vi "CRYSet Graph Title.vi"(8 "Inserted Graph VIRef out":refnum<vi>, 9 "Frame VIRef":refnum<vi>, 10 "Title State":bool, 11 "Title Name in":string) -> (3 "Title Name out":string)   [LabVIEW 2013]
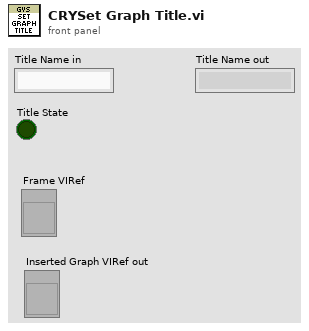
[diagram p1: front panel]
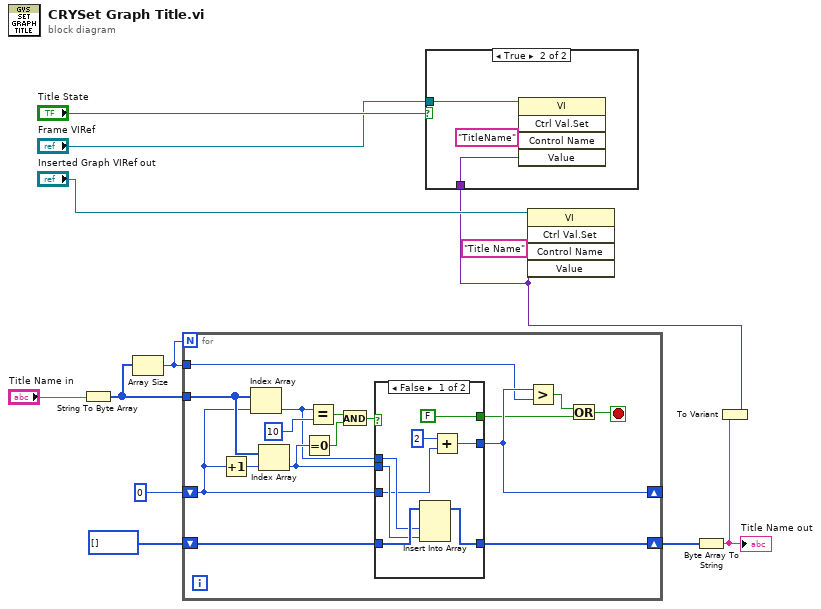
[diagram p0: block diagram]
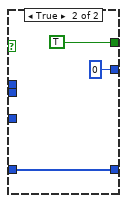
[diagram p3: hidden frame]
diagram:
  n1 = String To Byte Array(string="Title Name in") -> (unsigned byte array=w11:u8[])
  n2 = Array Size(array=w11) -> (size(s)=w9:i32)
  n3 = for {
    N: w9 -> [_]
    tunnel: w11 -> [w27]
    shift-right: [w19] -> w8
    shift-left: u8[] [] ("unsigned byte array") -> [w22]
    shift-right: [w17] -> _
    shift-left: 0 -> [w18]
    tunnel: w9 -> [w16]
    stop <- w13 stop-if-true
    n4 = Increment(x=w18) -> (x+1=w28:i32)
    n5 = Index Array(array=w27, index=w18) -> (element=w20:u8)
    n6 = Index Array(array=w27, index=w28) -> (element=w21:u8)
    n7 = Equal To 0?(x=w21) -> (x = 0?=w24:bool)
    n8 = Equal?(x=w20, y=u8 10) -> (x = y?=w23:bool)
    n9 = And(x=w23, y=w24) -> (x .and. y?=w25:bool)
    n10 = case shown="False" w25 {
      tunnel: [FALSE TRUE] -> w14
      tunnel: w22 -> [w35 w38]
      tunnel: w21 -> [w33 _]
      tunnel: w20 -> [w34 _]
      tunnel: [w32 w38] -> w19
      tunnel: [w31 0] -> w17
      tunnel: w18 -> [w30 _]
      frame False {
        n11 = Insert Into Array(array=w35, new element #1=w34, new element #2=w33) -> (w32:u8[])  [unwired: 1 in]
        n12 = Add(x=2, y=w30) -> (x+y=w31:i32)
      }
      frame True {
      }
    }
    n13 = Greater?(x=w17, y=w16) -> (0:w15:bool)
    n14 = Or(x=w15, y=w14) -> (x .or. y?=w13:bool)
  }
  n15 = Byte Array To String(unsigned byte array=w8) -> (string=w2:string)
  "Title Name out" <- w2
  n16 = To Variant(anything=w2) -> (Variant=w1:variant)
  n17 = case shown="True" "Title State" {
    tunnel: "Frame VIRef" -> [_ w41]
    tunnel: w1 -> [_ w40]
    frame False {
    }
    frame True {
      n18 = invoke class="VI" method="Ctrl Val.Set"(reference=w41, "Control Name"="TitleName", "Value"=w40) -> ()  [unwired: 2 in, 5 out]
    }
  }
  n19 = invoke class="VI" method="Ctrl Val.Set"(reference="Inserted Graph VIRef out", "Control Name"="Title Name", "Value"=w1) -> ()  [unwired: 2 in, 5 out]
